vi "Configuration-Global.vi"() -> ()   [LabVIEW 2014]
panel:
  in  "COM":string
  in  "IPC_6220_TCP_Port":i32
  in  "Terminal_UDP_Port":i32
  in  "IPC_UDP_Port":i32
  in  "IPC_Modbus_Port":i32
  in  "Terminal_IP":string
  in  "IPC_IP":string
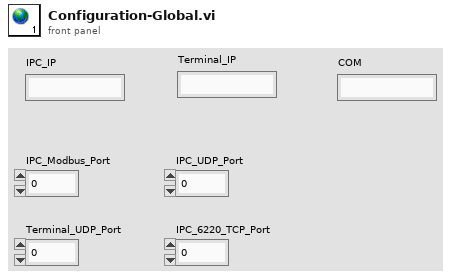
[diagram p1: front panel]
diagram:
